vi "Buffer Connections List_Initialize.vi"(8 "error in (no error)":errorcluster) -> (0 "error out":errorcluster {"code" min=0 max=0}, 3 "Connections Ref":T1)   [LabVIEW 2013, in "J1939 Addon Engine.lvlib"]
uses:
  Engine/J1939 Addon Engine.lvlib
  Types/BAM Buffer Connections List_Ref.ctl
  Types/TP Buffer Connection Cluster.ctl
  Types/TP Connections List State.ctl
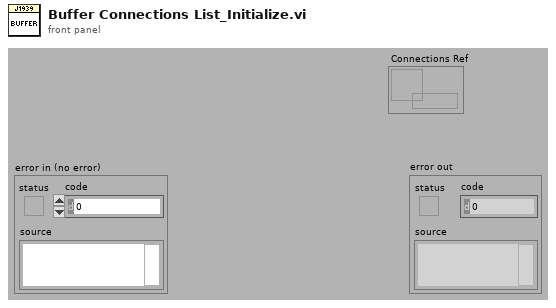
[diagram p1: front panel]
types:
  T1 = typedef "J1939 Addon Engine.lvlib/BAM Buffer Connections List_Ref.ctl" = refnum<data-value>
  T2 = typedef "J1939 Addon Engine.lvlib/TP Buffer Connection Cluster.ctl" = cluster{"Source Address":u8, "Destination Address":u8, "PGN":u32, "Arb ID":u32, "CAN Conversion Index":u32, "Total Expected Bytes":u16, "Total Expected Packets":u8, "Number of Packets Read":u8, "Start Time":u32, "Packets (U8)":u8[], "Timestamp":timestamp}
  T3 = typedef "J1939 Addon Engine.lvlib/TP Connections List State.ctl" = enum16{"Add", "Update", "Get", "Remove", "Initialize"}
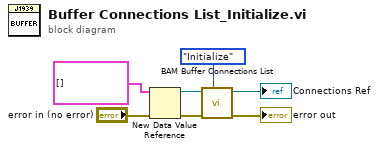
[diagram p0: block diagram]
diagram:
  n1 = New Data Value Reference(data value=T2[] [] ("Connections"), error in="error in (no error)") -> (data value reference=w4:refnum<data-value>, error out=w5:errorcluster)
  n2 = call "BAM Buffer Connections List.vi"("State"=TP_Connections_List_State."Initialize", "error in (no error)"=w5, "Connections Ref"=w4) -> ("error out"=→"error out":errorcluster, "Connections Ref out"=→"Connections Ref":T1)  [unwired: 5 in, 2 out]
